vi "Demo.vi"() -> ()   [LabVIEW 2015]
uses:
  MyGraph.xctl
  <vilib>/measure/NI_MABase.lvlib
panel:
  out "MyGraph":waveform(dbl)[](xcontrol)
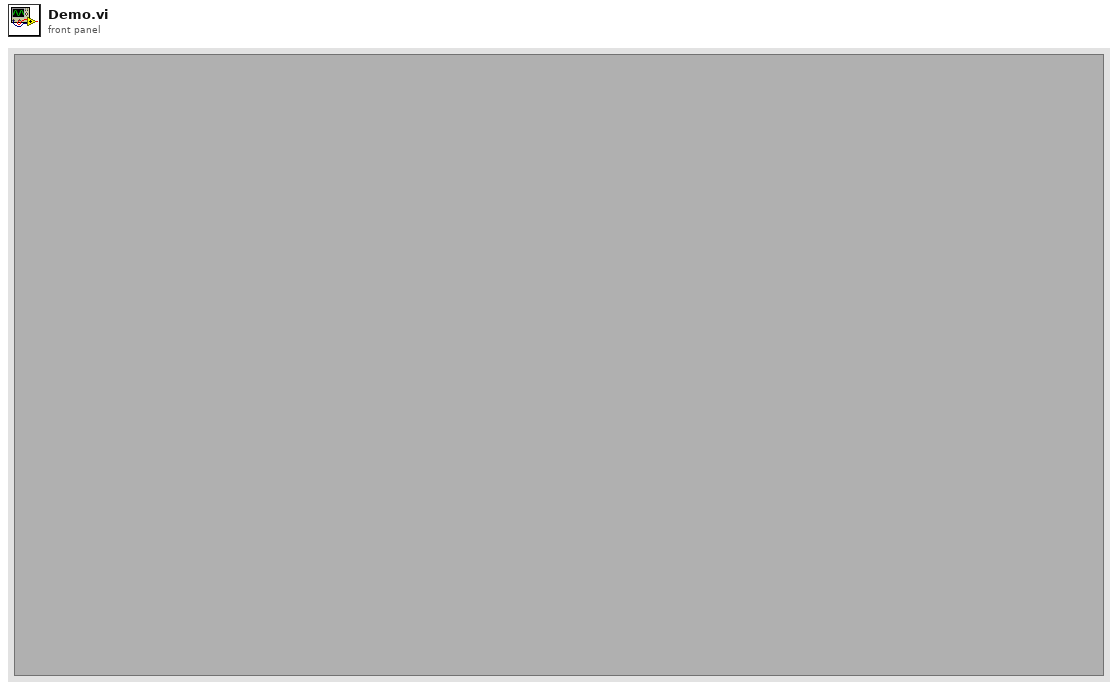
[diagram p1: front panel]
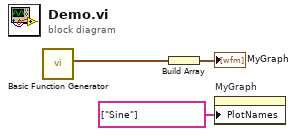
[diagram p0: block diagram]
diagram:
  n1 = call <vilib>:"Basic Function Generator.vi"() -> ("signal out"=w3:waveform(dbl))  [unwired: 9 in, 2 out]
  n2 = Build Array(w3) -> (→"MyGraph":waveform(dbl)[])
  n3 = property on="MyGraph" class="MyGraph (strict)"("PlotNames"=string[] ["Sine"]) -> ()  [unwired: 2 in, 2 out]
